vi "Autonomous Encoder2 Read.vi"(8 "error in (no error)":errorcluster) -> (0 "error out":errorcluster, 1 "Encoder Direction":string, 2 "Encoder Distance":dbl)   [LabVIEW 2016]
panel:
  out "Encoder Rate":dbl
  out "Encoder State":string
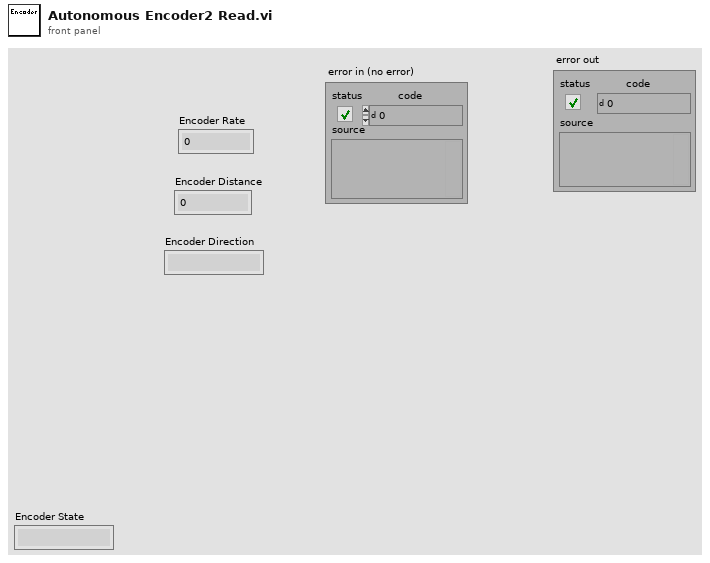
[diagram p1: front panel]
types:
  T1 = typedef "WPI_EncoderDevRef.ctl" = cluster{"DevStatus":errorcluster, "EncoderIndex":T2, "CounterIndex":T3, "DistancePerCount":dbl, "Decoding Type":T4}
  T2 = typedef "FPGA_EncoderIdx.ctl" = enum8{"Enc 0", "Enc 1", "Enc 2", "Enc 3", "Enc 4", "Enc 5", "Enc 6", "Enc 7", "Invalid"}
  T3 = typedef "FPGA_CounterCtrSystemIndex.ctl" = enum8{"Ctr 0", "Ctr 1", "Ctr 2", "Ctr 3", "Ctr 4", "Ctr 5", "Ctr 6", "Ctr 7", "Invalid"}
  T4 = typedef "WPI_EncoderType.ctl" = enum16{"1x", "2x", "4x"}
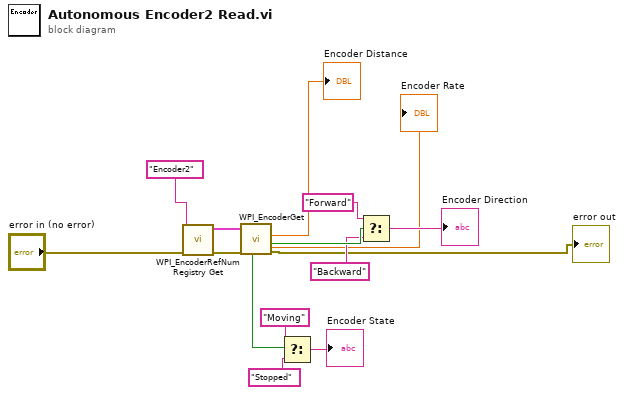
[diagram p0: block diagram]
diagram:
  n1 = call <vilib>:"WPI_EncoderRefNum Registry Get.vi"("error in (no error)"="error in (no error)", "refnum name"="Encoder2") -> ("error out"=w14:errorcluster, "EncoderDevRef"=w15:T1)  [unwired: 8 in]
  n2 = call <vilib>:"WPI_EncoderGet.vi"("error in (no error)"=w14, "EncoderDevRef"=w15) -> ("error out"=→"error out":errorcluster, "Direction"=w11:bool, "Distance"=→"Encoder Distance":dbl, "Rate"=→"Encoder Rate":dbl, "Stopped"=w12:bool)  [unwired: 4 in, 1 out]
  n3 = Select(t="Moving", s=w12, f="Stopped") -> (s? t:f=→"Encoder State":string)
  n4 = Select(t="Forward", s=w11, f="Backward") -> (s? t:f=→"Encoder Direction":string)
